vi "UDP - Find UDP Broadcast IPs.vi"() -> (3 "IP Addresses":u32[](array[numeric]))   [LabVIEW 2021]
doc: "List all IP addresses on the local computer.\nSet the last number in the IP address to 255.\nSo, 192.168.1.1 becomes 192.168.1.255\nBroadcasting to 192.168.1.255 will comunicate with all devices\nin the range of 192.168.1.x"
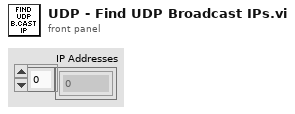
[diagram p1: front panel]
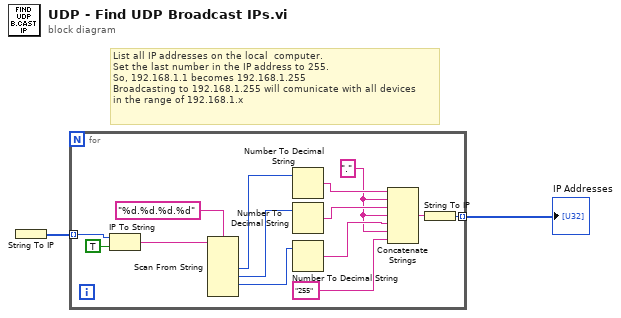
[diagram p0: block diagram]
diagram:
  # "List all IP addresses on the local  computer.\nSet the last number in the IP address to 255.\nSo, 192.168.1.1 becomes 192.168.1.255\nBroadcasting to 192.168.1.255 will comunicate with all devices\nin the range of 192.168.1.x"
  n1 = String To IP() -> (0:w1:u32[])  [unwired: 1 in]
  n2 = for {
    tunnel: w1 -> [w15] mode=indexing
    tunnel: [w3] -> w2 mode=indexing
    w6 = "." ("string")
    n3 = IP To String(1:TRUE ("dot notation? (F)"), 2:w15) -> (0:w14:string)
    n4 = Scan From String(format string="%d.%d.%d.%d", input string=w14) -> (output 1=w12:i32, output 2=w11:i32, output 3=w10:i32)  [unwired: 7 in, 3 out]
    n5 = Number To Decimal String(number=w12) -> (decimal integer string=w9:string)  [unwired: 1 in]
    n6 = Number To Decimal String(number=w11) -> (decimal integer string=w8:string)  [unwired: 1 in]
    n7 = Number To Decimal String(number=w10) -> (decimal integer string=w7:string)  [unwired: 1 in]
    n8 = Concatenate Strings(w9, w6, w8, w6, w7, w6, "255" ("string")) -> (w4:string)
    n9 = String To IP(1:w4) -> (0:w3:u32)
  }
  "IP Addresses" <- w2
